vi "pict.Draw.RGB.vi"(6 "top-left (0,0)":T1, 9 "RGB pixmap":u32[][](array[numeric]) format="%06x") -> (1 "picture":picture)   [LabVIEW 2020]
uses:
  <vilib>/Utility/miscctls.llb/LVPositionTypeDef.ctl
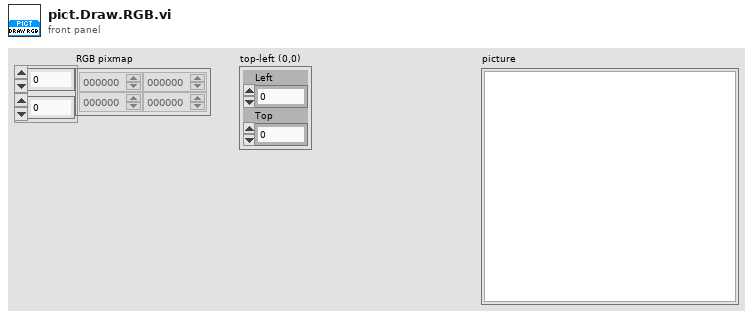
[diagram p1: front panel]
types:
  T1 = typedef "LVPositionTypeDef.ctl" = cluster{"Left":i32, "Top":i32}
  T2 = cluster{"top":i16, "left":i16, "bottom":i16, "right":i16}
  T3 = cluster{"default foreground":u32, "default background":u32}
  T4 = cluster{"opcode":i16, i32, i32, "Rectangle":cluster{"top":i16, "left":i16, "bottom":i16, "right":i16}, "bit depth":i16, cluster{"default foreground":u32, "default background":u32}}
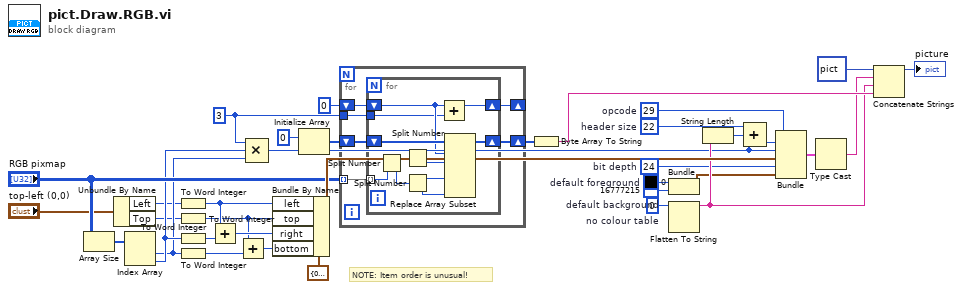
[diagram p0: block diagram]
diagram:
  w15 = 3 ("y")
  w27 = i16 0  # no colour table
  w20 = i16 24  # bit depth
  w24 = u32 16777215  # default background
  w28 = u32 0  # default foreground
  w33 = 22  # header size
  w34 = i16 29  # opcode
  # "NOTE: Item order is unusual!"
  n1 = Array Size(array="RGB pixmap") -> (size(s)=w18:i32[])
  n2 = Unbundle By Name("top-left (0,0)") -> ("Left"=w4:i32, "Top"=w2:i32)
  n3 = Index Array(array=w18) -> (element #1=w9:i32, element #2=w10:i32)  [unwired: 2 in]
  n4 = To Word Integer(number=w4) -> (16bit integer=w3:i16)
  n5 = To Word Integer(number=w2) -> (16bit integer=w1:i16)
  n6 = To Word Integer(number=w10) -> (16bit integer=w7:i16)
  n7 = To Word Integer(number=w9) -> (16bit integer=w6:i16)
  n8 = Add(x=w3, y=w7) -> (x+y=w12:i16)
  n9 = Add(x=w1, y=w6) -> (x+y=w11:i16)
  n10 = Compound Arithmetic op=MULTIPLY(w15, w10, w9) -> (w16:i32)
  n11 = Bundle By Name(cluster=T2 {"top"=0, "left"=0, "bottom"=0, "right"=0} ("Rectangle"), "left"=w3, "top"=w1, "right"=w12, "bottom"=w11) -> (w30:T2)
  n12 = Initialize Array(u8 0 ("element"), w16) -> (w19:u8[])
  n13 = for {
    tunnel: "RGB pixmap" -> [w41] mode=indexing
    shift-right: [w42] -> w35
    shift-left: w19 -> [w40]
    shift-right: [w39] -> _
    shift-left: 0 -> [w38]
    tunnel: w15 -> [w37]
    n14 = for {
      tunnel: w41 -> [w49] mode=indexing
      shift-right: [w52] -> w42
      shift-left: w40 -> [w53]
      shift-right: [w51] -> w39
      shift-left: w38 -> [w50]
      tunnel: w37 -> [w43]
      n15 = Split Number(x=w49) -> (hi(x)=w46:u16, lo(x)=w48:u16)
      n16 = Split Number(x=w46) -> (lo(x)=w44:u8)  [unwired: 1 out]
      n17 = Split Number(x=w48) -> (hi(x)=w45:u8, lo(x)=w47:u8)
      n18 = Add(x=w50, y=w43) -> (x+y=w51:i32)
      n19 = Replace Array Subset(array=w53, new element #1=w44, index #1=w50, new element #2=w45, new element #3=w47) -> (w52:u8[])  [unwired: 2 in]
    }
  }
  n20 = Byte Array To String(unsigned byte array=w35) -> (string=w31:string)
  n21 = Bundle("default foreground"=w28, "default background"=w24) -> (w25:T3)  [unwired: 1 in]
  n22 = Flatten To String(anything=w27) -> (data string=w26:string)  [unwired: 3 in, 2 out]
  n23 = String Length(string=w26) -> (length=w29:i32)
  n24 = Compound Arithmetic op=ADD(w33, w29, w16) -> (w32:i32)
  n25 = Bundle("opcode"=w34, w32, w16, "Rectangle"=w30, "bit depth"=w20, w25) -> (w21:T4)  [unwired: 1 in]
  n26 = Type Cast(x=w21) -> (*(type *) &x=w23:string)  [unwired: 1 in]
  n27 = Concatenate Strings(picture data[5B] ("new picture"), w23, w26, w31) -> (→"picture":picture)
